vi "AdjustTurning.vi"(10 "Speed":dbl, 11 "ZAxisInput":dbl) -> (3 "ZAxisOutput":dbl)   [LabVIEW 2017]
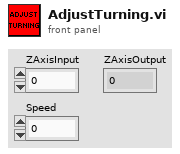
[diagram p1: front panel]
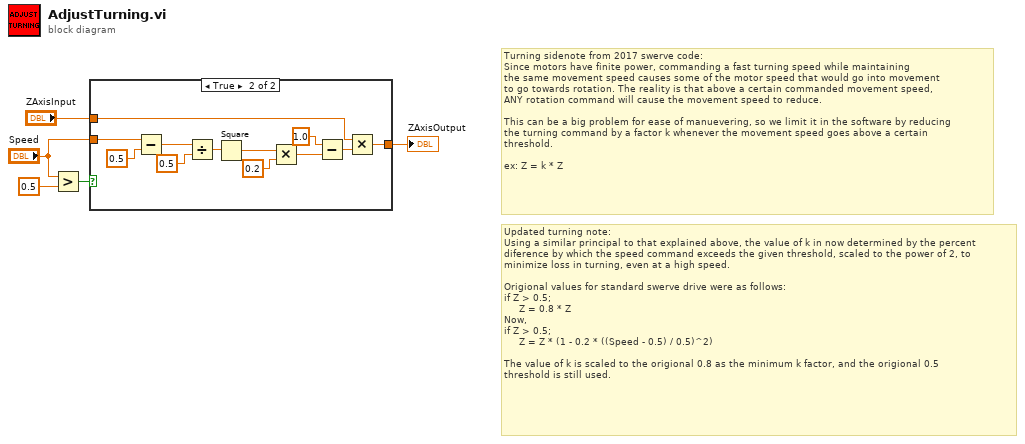
[diagram p0: block diagram]
diagram:
  # "Updated turning note:\nUsing a similar principal to that explained above, the value of k in now determined by the percent\ndiference by which the speed command exceeds the given threshold, scaled to the power of 2, to\nminimize loss in turning, even at a high speed.\n\nOrigional values for standard swerve drive were as follows:\nif Z > 0.5;\n     Z = 0.8 * Z\nNow,\nif Z > 0.5;\n     Z = Z * (1 - 0.2 * ((Speed - 0.5) / 0.5)^2)\n\nThe value of k is scaled to the origional 0.8 as the minimum k factor, and the origional 0.5\nthreshold is still used."
  # "Turning sidenote from 2017 swerve code:\nSince motors have finite power, commanding a fast turning speed while maintaining\nthe same movement speed causes some of the motor speed that would go into movement\nto go towards rotation. The reality is that above a certain commanded movement speed,\nANY rotation command will cause the movement speed to reduce.\n\nThis can be a big problem for ease of manuevering, so we limit it in the software by reducing\nthe turning command by a factor k whenever the movement speed goes above a certain\nthreshold.\n\nex: Z = k * Z"
  n1 = Greater?(x="Speed", y=0.5) -> (0:w4:bool)
  n2 = case shown="True" w4 {
    tunnel: "ZAxisInput" -> [w6 w13]
    tunnel: [w6 w14] -> w2
    tunnel: "Speed" -> [_ w18]
    frame False {
    }
    frame True {
      n3 = Subtract(x=w18, y=0.5) -> (x-y=w16:dbl)
      n4 = Divide(x=w16, y=0.5) -> (x/y=w7:dbl)
      n5 = Square(x=w7) -> (x^2=w12:dbl)
      n6 = Multiply(x=w12, y=0.2) -> (x*y=w10:dbl)
      n7 = Subtract(x=1.0, y=w10) -> (x-y=w8:dbl)
      n8 = Multiply(x=w13, y=w8) -> (x*y=w14:dbl)
    }
  }
  "ZAxisOutput" <- w2
